vi "Get ControllerIP.vi"(8 "error in (no error)":errorcluster, 11 "Device Item Ref in":T1 format="%.0x") -> (0 "error out":errorcluster, 2 "element":string, 3 "Device Item Ref out":T1 format="%.0x")   [LabVIEW 2018, in "CAN Gateway System Explorer.lvlib"]
uses:
  CAN Gateway System Explorer.lvlib
  <vilib>/NI Veristand/Custom Device API/Custom Device Item Ref.ctl
  NationalInstruments.VeriStand.SystemDefinitionAPI
  <vilib>/NI Veristand/Custom Device Tools/Custom Device Utility Library/Custom Device Utility Library.lvlib
  <vilib>/NI Veristand/Custom Device API/Custom Device API.lvlib
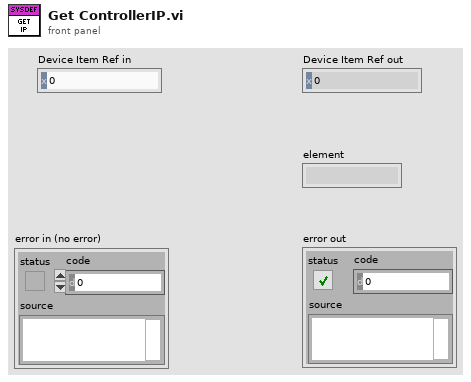
[diagram p1: front panel]
types:
  T1 = typedef "Custom Device API.lvlib/Custom Device Item Ref.ctl" = u64
  T2 = typedef "Custom Device API.lvlib/Custom Device Item Info.ctl" = cluster{"Name":string, "Is Channel":bool, "GUID":string, "Is Waveform":bool}
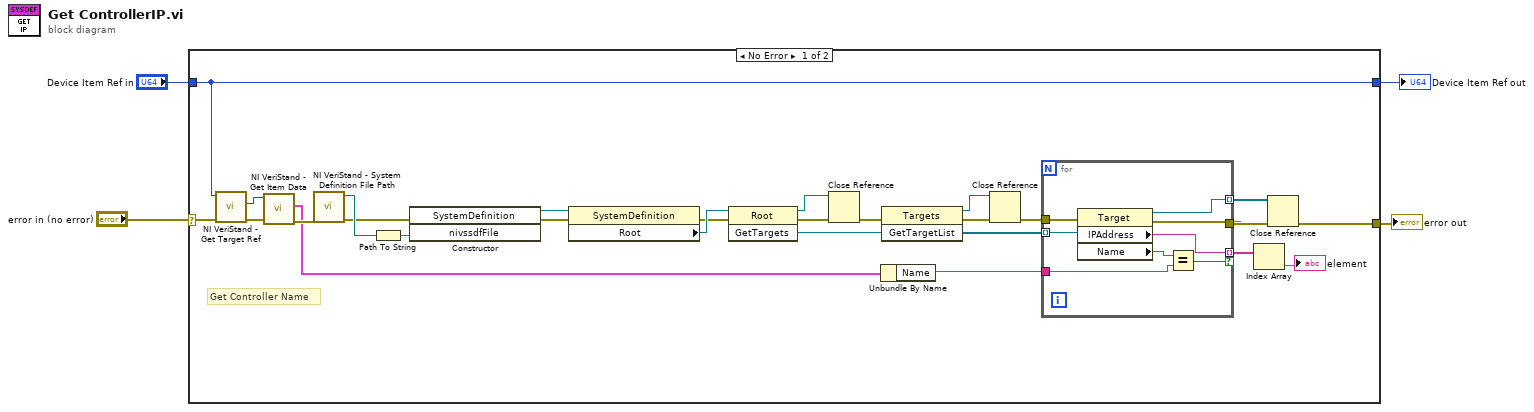
[diagram p0: block diagram]
diagram:
  n1 = case shown="No Error" "error in (no error)" {
    selector: "error in (no error)" -> [w15 w40]
    tunnel: "Device Item Ref in" -> [w8 w41]
    tunnel: [w8 w41] -> w2
    tunnel: [w7 w40] -> w1
    frame No Error {
      # "Get Controller Name"
      n2 = call <vilib>:"NI VeriStand - Get Target Ref.vi"("error in"=w15, "Item Ref in"=w8) -> ("error out"=w13:errorcluster, "Target Ref"=w9:T1)  [unwired: 6 in, 2 out]
      n3 = call <vilib>:"NI VeriStand - Get Item Data.vi"("error in (no error)"=w13, "Item Ref in"=w9) -> ("error out"=w12:errorcluster, "Item Info"=w11:T2)  [unwired: 6 in, 2 out]
      n4 = call <vilib>:"NI VeriStand - System Definition File Path.vi"("error in (no error)"=w12) -> ("error out"=w22:errorcluster, "SDF path"=w23:path)  [unwired: 9 in]
      n5 = Path To String(path=w23) -> (string=w24:string)
      n6 = constructor class="SystemDefinition"(error in=w22, "nivssdfFile"=w24) -> (reference out=w31:refnum<k24>, error out=w25:errorcluster)  [unwired: 2 in, 2 out]
      n7 = property class="SystemDefinition"(reference=w31, error in=w25) -> (error out=w26:errorcluster, "Root"=w30:refnum<k24>)  [unwired: 1 out]
      n8 = invoke class="Root" method="GetTargets"(reference=w30, error in=w26) -> (reference out=w29:refnum<k24>, error out=w27:errorcluster, "GetTargets"=w28:refnum<k24>)  [unwired: 1 in]
      n9 = Close Reference(reference=w29, error in (no error)=w27) -> (error out=w18:errorcluster)
      n10 = Unbundle By Name(w11) -> ("Name"=w14:string)
      n11 = invoke class="Targets" method="GetTargetList"(reference=w28, error in=w18) -> (reference out=w20:refnum<k24>, error out=w19:errorcluster, "GetTargetList"=w21:refnum<k24>[])  [unwired: 1 in]
      n12 = Close Reference(reference=w20, error in (no error)=w19) -> (error out=w16:errorcluster)
      n13 = for {
        tunnel: w21 -> [w39] mode=indexing
        tunnel: [w38] -> w6 mode=indexing if=w35
        tunnel: [w37] -> w17 mode=indexing
        tunnel: w16 -> [w34]
        tunnel: [w33] -> w10
        tunnel: w14 -> [w32]
        n14 = property class="Target"(reference=w39, error in=w34) -> (reference out=w37:refnum<k24>, error out=w33:errorcluster, "IPAddress"=w38:string, "Name"=w36:string)
        n15 = Equal?(x=w36, y=w32) -> (x = y?=w35:bool)
      }
      n16 = Index Array(array=w6) -> (element=→"element":string)  [unwired: 1 in]
      n17 = Close Reference(reference=w17, error in (no error)=w10) -> (error out=w7:errorcluster)
    }
    frame Error {
    }
  }
  "Device Item Ref out" <- w2
  "error out" <- w1
